vi "Read DVR.vi"(0 "Stop":bool, 7 "Get Data":bool, 11 "Error in":errorcluster) -> (15 "Error out":errorcluster)   [LabVIEW 2020, in "DVR Handson.lvlib"]
uses:
  DVR Handson.lvlib
  Typedefs/LV2 Operations.ctl
panel:
  out "data value":dbl
  # "GET DVR REFRENCE"
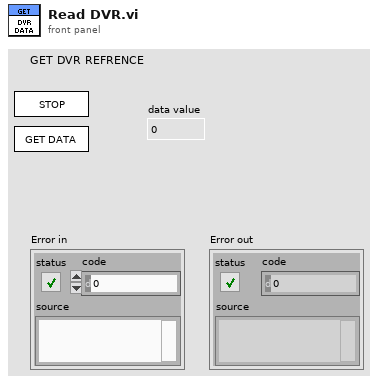
[diagram p1: front panel]
types:
  T1 = typedef "DVR Handson.lvlib/LV2 Operations.ctl" = enum16{"Initialize", "Read", "Write"}
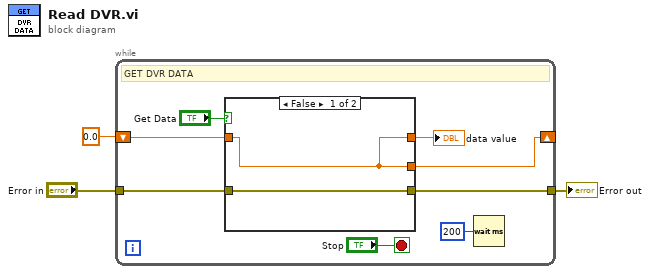
[diagram p0: block diagram]
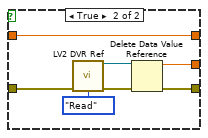
[diagram p2: hidden frame]
diagram:
  n1 = while {
    tunnel: "Error in" -> [w9]
    tunnel: [w6] -> w2
    shift-right: [w8] -> _
    shift-left: 0.0 -> [w7]
    stop <- "Stop" stop-if-true
    # "GET DVR DATA"
    n2 = case shown="False" "Get Data" {
      tunnel: w9 -> [w13 w20]
      tunnel: [w13 w17] -> w6
      tunnel: [w12 w15] -> w8
      tunnel: w7 -> [w12 w14]
      tunnel: [w12 w14] -> w4
      frame False {
      }
      frame True {
        n3 = call "LV2 DVR Ref.vi"("Error in"=w20, "Operation"=LV2_Operations."Read") -> ("DVR Output"=w16:refnum<data-value>, "Error out"=w18:errorcluster)  [unwired: 12 in]
        n4 = Delete Data Value Reference(data value reference=w16, error in=w18) -> (data value=w15:dbl, error out=w17:errorcluster)
      }
    }
    "data value" <- w4
    n5 = Wait (ms)(milliseconds to wait=u32 200) -> ()  [unwired: 1 out]
  }
  "Error out" <- w2
